vi "MPB_save_test_results.vi"(9 "test results array":T1[](array[typedef]), 10 "filename":path=path "Example Tab-Delimited File.txt", 11 "base path":path) -> ()   [LabVIEW 2020]
uses:
  controls/test results.ctl
  controls/MPB_step_type.ctl
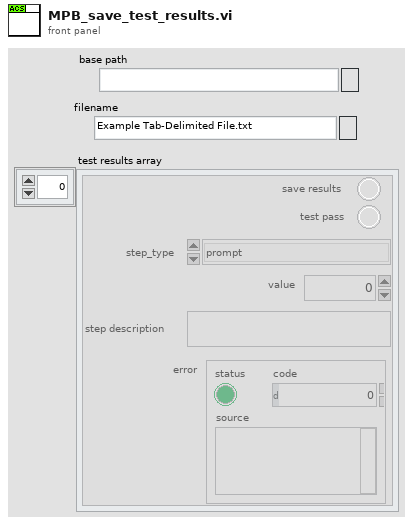
[diagram p1: front panel]
types:
  T1 = typedef "test results.ctl" = cluster{"test pass":bool, "step_type":T2, "value":dbl, "step description":string, "error":errorcluster, "save results":bool}
  T2 = typedef "MPB_step_type.ctl" = enum16{"default", "prompt", "sequence#", "12V_1_power supply on_off", "12V_2_power supply on_off", "set_hipot_V", "set_hipot_I_limit", "set_hipot_ramping (sec)", "set hipot_hold_time", "read_hipot_V", "read_hipot_I", "set_daq", "read_daq", "flash uds", "wait (sec)", "record_pass_fail", "ac_charge_test", "dc_400V_charging", "HAPS Heater Output", "HAPS Compressor Output", "abort_test", "end_of_test", "error_exit"}
  T3 = enum16{"open", "replace", "create", "open or create", "replace or create", "replace or create with confirmation"}
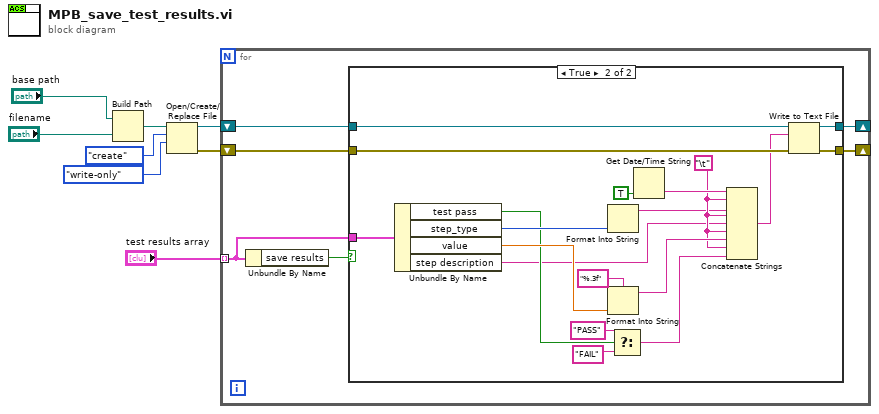
[diagram p0: block diagram]
diagram:
  n1 = Build Path(base path="base path", name or relative path="filename") -> (appended path=w5:path)
  n2 = Open/Create/Replace File(file path (use dialog)=w5, operation (0:open)=T3."create", access (0:read/write)=enum16{"read/write", "read-only", "write-only"}."write-only") -> (refnum out=w3:refnum<file>, error out=w2:errorcluster)  [unwired: 1 in, 3 out]
  n3 = for {
    tunnel: "test results array" -> [w13] mode=indexing
    shift-right: [w10] -> _
    shift-left: w3 -> [w12]
    shift-right: [w9] -> _
    shift-left: w2 -> [w11]
    n4 = Unbundle By Name(w13) -> ("save results"=w14:bool)
    n5 = case shown="True" w14 {
      tunnel: w13 -> [_ w35]
      tunnel: w12 -> [w16 w20]
      tunnel: w11 -> [w15 w21]
      tunnel: [w16 w18] -> w10
      tunnel: [w15 w17] -> w9
      frame False {
      }
      frame True {
        w28 = "\t" ("Tab")
        n6 = Unbundle By Name(w35) -> ("test pass"=w27:bool, "step_type"=w32:T2, "value"=w31:dbl, "step description"=w22:string)
        n7 = Format Into String(w32) -> (resulting string=w23:string)  [unwired: 3 in, 1 out]
        n8 = Format Into String(format string="%.3f", w31) -> (resulting string=w30:string)  [unwired: 2 in, 1 out]
        n9 = Select(t="PASS", s=w27, f="FAIL") -> (s? t:f=w24:string)
        n10 = Get Date/Time String(want seconds? (F)=TRUE) -> (time string=w34:string)  [unwired: 2 in, 1 out]
        n11 = Concatenate Strings(w34, w28, w23, w28, w22, w28, w30, w28, w24) -> (w19:string)
        n12 = Write to Text File(file (use dialog)=w20, text=w19, error in=w21) -> (refnum out=w18:refnum<file>, error out=w17:errorcluster)  [unwired: 1 in, 1 out]
      }
    }
  }
